vi "Get State Value Index.vi"(8 "error in (no error)":errorcluster, 9 "Channel Name":string, 10 "State Value":dbl, 11 "State Value Array":i32[](array[numeric])) -> (0 "error out":errorcluster, 3 "index of element":i32)   [LabVIEW 2020, in "Routing and Faulting Shared.lvlib"]
uses:
  Dependencies.llb/Routing and Faulting Shared.lvlib
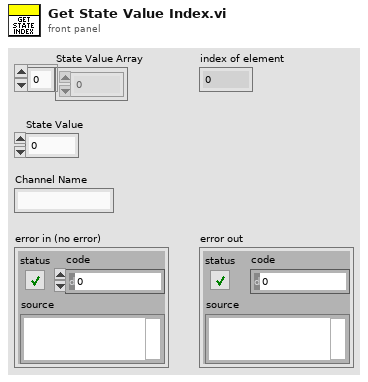
[diagram p1: front panel]
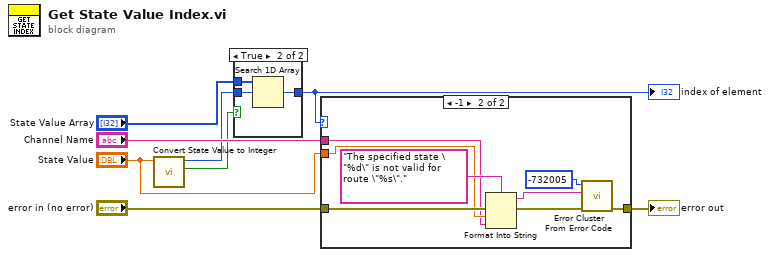
[diagram p0: block diagram]
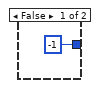
[diagram p3: hidden frame]
diagram:
  n1 = call "Convert State Value to Integer.vi"("Floating Point State Value"="State Value") -> ("Valid State Value"=w1:bool, "Integer State Value"=w3:i32)  [unwired: 9 in]
  n2 = case shown="True" w1 {
    tunnel: w3 -> [_ w12]
    tunnel: [-1 ("index of element") w10] -> w4
    tunnel: "State Value Array" -> [_ w11]
    frame False {
    }
    frame True {
      n3 = Search 1D Array(1D array=w11, element=w12) -> (index of element=w10:i32)  [unwired: 1 in]
    }
  }
  "index of element" <- w4
  n4 = case shown="-1" w4 {
    tunnel: "error in (no error)" -> [w13 w17]
    tunnel: [w13 w16] -> w6
    tunnel: "State Value" -> [_ w15]
    tunnel: "Channel Name" -> [_ w14]
    frame Default {
    }
    frame -1 {
      n5 = Format Into String(format string="The specified state \"%d\" is not valid for route \"%s\".", error in=w17, w15, w14) -> (resulting string=w20:string, error out=w19:errorcluster)  [unwired: 1 in]
      n6 = call <vilib>:"Error Cluster From Error Code.vi"("error in (no error)"=w19, "error message (\"\")"=w20, "error code (0)"=-732005) -> ("error out"=w16:errorcluster)  [unwired: 6 in]
    }
  }
  "error out" <- w6
